vi "SetParam.vi"(8 "error in (no error)":errorcluster caption="entrée d'erreur (pas d'erreur)", 10 "DictVectorizer":T1={"dtype"="float", "separator"="=", "sparse"=TRUE, "sort"=TRUE}, 11 "DictVectorizer.lvclass":refnum<class "DictVectorizer.lvclass">) -> (0 "error out":errorcluster caption="sortie d'erreur", 3 "DictVectorizer.lvclass":refnum<class "DictVectorizer.lvclass">)   [LabVIEW 2020, in "DictVectorizer.lvclass"]
doc: "Set Parameters"
uses:
  DictVectorizer.lvclass
  DictVectorizer.lvclass/DictVectorizer.ctl
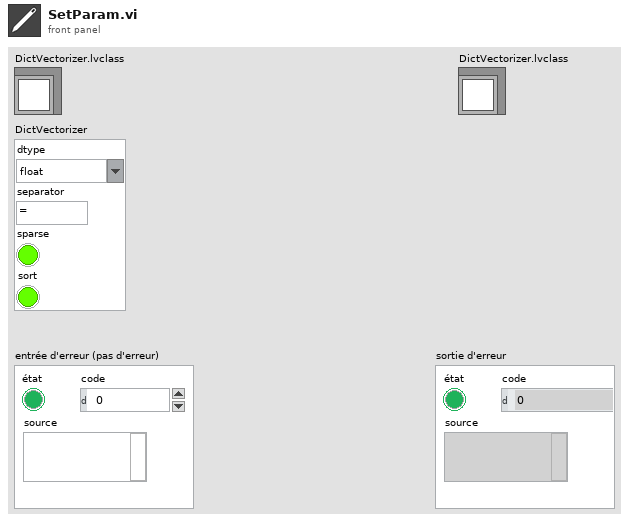
[diagram p1: front panel]
types:
  T1 = cluster{"dtype":string, "separator":string, "sparse":bool, "sort":bool}
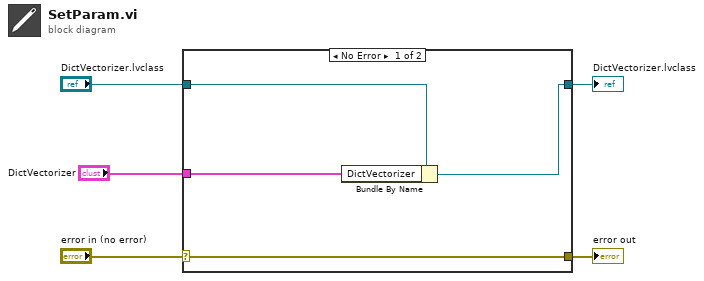
[diagram p0: block diagram]
diagram:
  n1 = case shown="No Error" "error in (no error)" {
    selector: "error in (no error)" -> [w9 w10]
    tunnel: [w9 w10] -> w4
    tunnel: [w7 w11] -> w2
    tunnel: "DictVectorizer.lvclass" -> [w8 w11]
    tunnel: "DictVectorizer" -> [w6 _]
    frame No Error {
      n2 = Bundle By Name(cluster=w8, "DictVectorizer"=w6) -> (w7:refnum<class "DictVectorizer.lvclass">)
    }
    frame Error {
    }
  }
  "error out" <- w4
  "DictVectorizer.lvclass" <- w2
